vi "Enable-Disable UI Elements.vi"(8 "error in (no error)":errorcluster, 9 "Enable/Disable":T1(ring), 11 "Ctrl ref's":refnum<vi>[](array[refnum])) -> (0 "error out":errorcluster)   [LabVIEW 2013]
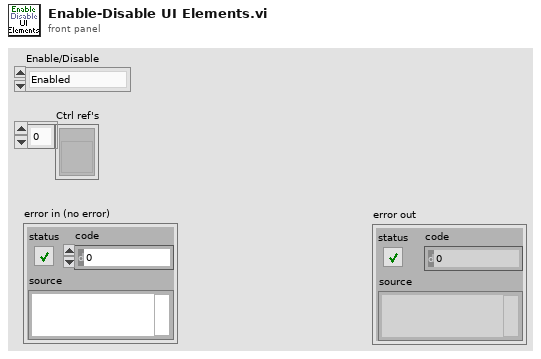
[diagram p1: front panel]
types:
  T1 = enum8{"Enabled", "Disabled", "Disabled and Grayed Out"}
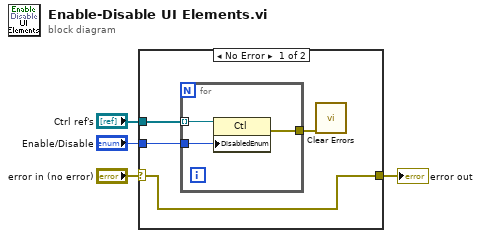
[diagram p0: block diagram]
diagram:
  n1 = case shown="No Error" "error in (no error)" {
    selector: "error in (no error)" -> [w5 w12]
    tunnel: "Enable/Disable" -> [w8 _]
    tunnel: "Ctrl ref's" -> [w7 _]
    tunnel: [w5 w12] -> w1
    frame No Error {
      n2 = for {
        tunnel: w7 -> [w11] mode=indexing
        tunnel: w8 -> [w10]
        tunnel: [w9] -> w6
        n3 = property on="Property Node" class="Ctl"(reference=w11, "DisabledEnum"=w10) -> (error out=w9:errorcluster)  [unwired: 1 in, 1 out]
      }
      n4 = call <vilib>:"Clear Errors.vi"("error in (no error)"=w6) -> ()  [unwired: 6 in, 1 out]
    }
    frame Error {
    }
  }
  "error out" <- w1
